vi "plugins_load.vi"(6 "Sub Panel":refnum<vi>, 7 "Plugin Chooser":refnum<vi>) -> (0 "error out":errorcluster, 1 "Plugins":T1(array[cluster]), 2 "Sub Panel Out":refnum<vi>, 3 "Plugin Chooser Out":refnum<vi>)   [LabVIEW 2015]
uses:
  red_tweezers_globals_INTERNAL_VOLATILE.vi
panel:
  out "file or folder exists?":bool
  out "Plugins Folder":path
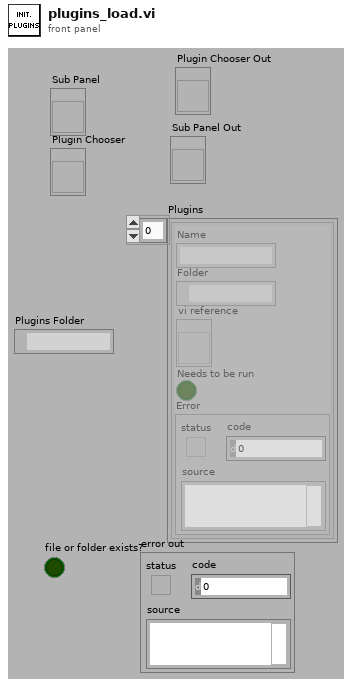
[diagram p1: front panel]
types:
  T1 = cluster{"Name":string, "Folder":path, "vi reference":refnum<vi>, "Needs to be run":bool, "Error":errorcluster}[]
  T2 = cluster{"Name":string, "Folder":path, "vi reference":refnum<vi>, "Needs to be run":bool, "Error":errorcluster}
  T3 = enum32{"Bad", "Idle", "Run top level", "Running"}
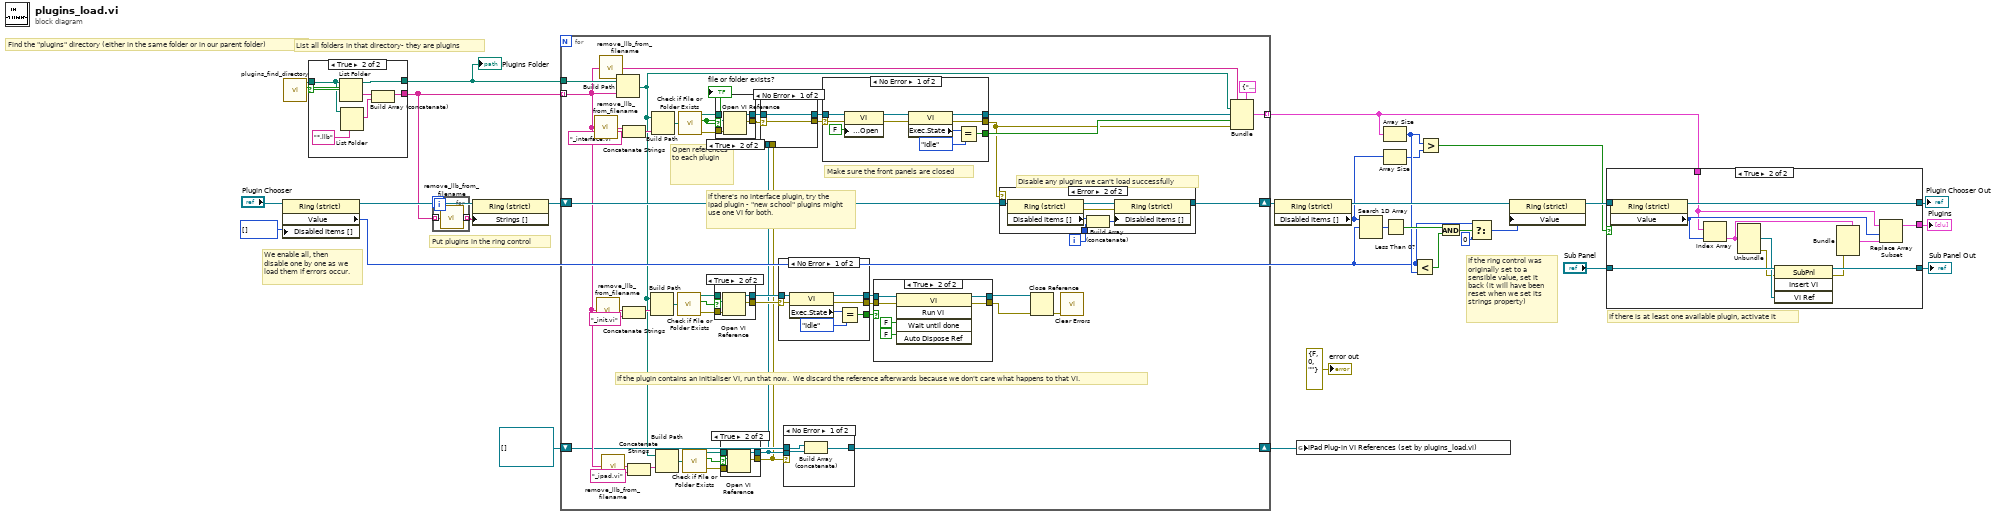
[diagram p0: block diagram]
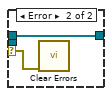
[diagram p4: hidden frame]
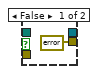
[diagram p5: hidden frame]
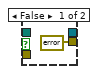
[diagram p7: hidden frame]
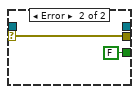
[diagram p8: hidden frame]
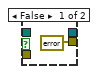
[diagram p10: hidden frame]
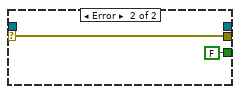
[diagram p11: hidden frame]
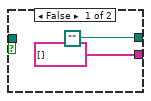
[diagram p12: hidden frame]
diagram:
  # "We enable all, then disable one by one as we load them if errors occur."
  # "If there is at least one available plugin, activate it"
  # "If the ring control was originally set to a sensible value, set it back (it will have been reset when we set its strings property)"
  # "Put plugins in the ring control"
  # "List all folders in that directory- they are plugins"
  # "Find the \"plugins\" directory (either in the same folder or in our parent folder)"
  n1 = property class="Ring (strict)"(reference="Plugin Chooser", "Disabled Items []"=i32[] []) -> (reference out=w25:refnum<vi>, "Value"=w4:u16)  [unwired: 1 in, 1 out]
  n2 = call "plugins_find_directory.vi"() -> ("file or folder exists?"=w30:bool, "dup path"=w31:path)  [unwired: 6 in]
  n3 = case shown="True" w30 {
    tunnel: w31 -> [_ w38]
    tunnel: [string[] [] ("folder names") w35] -> w9
    tunnel: [path "" w39] -> w29
    frame False {
    }
    frame True {
      n4 = List Folder(path=w38) -> (path out=w39:path, folder names=w36:string[])  [unwired: 3 in, 2 out]
      n5 = List Folder(path=w38, pattern="*.llb") -> (filenames=w34:string[])  [unwired: 2 in, 3 out]
      n6 = Build Array (concatenate)(w36, w34) -> (w35:string[])
    }
  }
  "Plugins Folder" <- w29
  n7 = for {
    tunnel: w9 -> [w41] mode=indexing
    tunnel: [w40] -> w8 mode=indexing
    n8 = call "remove_llb_from_filename.vi"("String"=w41) -> ("result string"=w40:string)
  }
  n9 = property class="Ring (strict)"(reference=w25, "Strings []"=w8) -> (reference out=w27:refnum<vi>)  [unwired: 1 in, 1 out]
  n10 = for {
    tunnel: w9 -> [w51] mode=indexing
    tunnel: w29 -> [w85]
    shift-right: [w80] -> w26
    shift-left: w27 -> [w81]
    tunnel: [w78] -> w19 mode=indexing
    shift-right: [w50] -> w2
    shift-left: refnum<vi>[] [] -> [w49]
    i -> [w82]
    # "if there's no interface plugin, try the ipad plugin - \"new school\" plugins might use one VI for both."
    # "If the plugin contains an initialiser VI, run that now.  We discard the reference afterwards because we don't care what happens to that VI."
    # "Open references to each plugin"
    # "Make sure the front panels are closed"
    # "Disable any plugins we can't load successfully"
    n11 = call "remove_llb_from_filename.vi"("String"=w51) -> ("result string"=w60:string)
    n12 = call "remove_llb_from_filename.vi"("String"=w51) -> ("result string"=w59:string)
    n13 = call "remove_llb_from_filename.vi"("String"=w51) -> ("result string"=w61:string)
    n14 = call "remove_llb_from_filename.vi"("String"=w51) -> ("result string"=w58:string)
    n15 = Build Path(base path=w85, name or relative path=w51) -> (appended path=w48:path)
    n16 = Concatenate Strings(w59, "_init.vi" ("string")) -> (w71:string)
    n17 = Concatenate Strings(w60, "_interface.vi" ("string")) -> (w90:string)
    n18 = Concatenate Strings(w58, "_ipad.vi" ("string")) -> (w54:string)
    n19 = Build Path(base path=w48, name or relative path=w71) -> (appended path=w63:path)
    n20 = Build Path(base path=w48, name or relative path=w90) -> (appended path=w88:path)
    n21 = Build Path(base path=w48, name or relative path=w54) -> (appended path=w57:path)
    n22 = call <vilib>:"Check if File or Folder Exists.vi"("path"=w63) -> ("error out"=w69:errorcluster, "file or folder exists?"=w75:bool, "dup path"=w72:path)  [unwired: 8 in]
    n23 = call <vilib>:"Check if File or Folder Exists.vi"("path"=w88) -> ("error out"=w83:errorcluster, "file or folder exists?"=w86:bool, "dup path"=w87:path)  [unwired: 8 in]
    "file or folder exists?" <- w86
    n24 = call <vilib>:"Check if File or Folder Exists.vi"("path"=w57) -> ("error out"=w56:errorcluster, "file or folder exists?"=w52:bool, "dup path"=w53:path)  [unwired: 8 in]
    n25 = case shown="True" w75 {
      tunnel: w72 -> [_ w117]
      tunnel: [_ w116] -> w73
      tunnel: [errorcluster {"status"=TRUE, "code"=0, "source"=""} ("error out") w115] -> w74
      tunnel: w69 -> [_ w114]
      frame False {
      }
      frame True {
        n26 = Open VI Reference(vi path=w117, error in (no error)=w114) -> (vi reference=w116:refnum<vi>, error out=w115:errorcluster)  [unwired: 4 in]
      }
    }
    n27 = case shown="True" w86 {
      tunnel: w87 -> [_ w139]
      tunnel: [_ w138] -> w46
      tunnel: [errorcluster {"status"=TRUE, "code"=0, "source"=""} ("error out") w137] -> w47
      tunnel: w83 -> [_ w136]
      frame False {
      }
      frame True {
        n28 = Open VI Reference(vi path=w139, error in (no error)=w136) -> (vi reference=w138:refnum<vi>, error out=w137:errorcluster)  [unwired: 4 in]
      }
    }
    n29 = case shown="True" w52 {
      tunnel: w53 -> [_ w104]
      tunnel: [_ w103] -> w44
      tunnel: [errorcluster {"status"=TRUE, "code"=0, "source"=""} ("error out") w102] -> w43
      tunnel: w56 -> [_ w101]
      frame False {
      }
      frame True {
        n30 = Open VI Reference(vi path=w104, error in (no error)=w101) -> (vi reference=w103:refnum<vi>, error out=w102:errorcluster)  [unwired: 4 in]
      }
    }
    n31 = case shown="No Error" w47 {
      selector: w47 -> [w91 _]
      tunnel: w46 -> [w92 _]
      tunnel: [w92 w94] -> w45
      tunnel: w44 -> [_ w94]
      tunnel: w43 -> [_ w93]
      tunnel: [w91 w93] -> w42
      frame No Error {
      }
      frame Error {
      }
    }
    n32 = case shown="No Error" w74 {
      selector: w74 -> [w119 w125]
      tunnel: w73 -> [w118 _]
      tunnel: [w124 _] -> w66
      tunnel: [w123 FALSE] -> w68
      tunnel: [w120 w125] -> w67
      frame No Error {
        n33 = property class="VI"(reference=w118, error in=w119) -> (reference out=w124:refnum<vi>, error out=w120:errorcluster, "Exec.State"=w122:T3)
        n34 = Equal?(x=w122, y=T3."Idle" ("Execution:State")) -> (x = y?=w123:bool)
      }
      frame Error {
      }
    }
    n35 = case shown="No Error" w43 {
      selector: w43 -> [_ w98]
      tunnel: w44 -> [w97 _]
      tunnel: [w96 w99] -> w50
      tunnel: w49 -> [w95 w99]
      frame No Error {
        n36 = Build Array (concatenate)(w95, w97) -> (w96:refnum<vi>[])
      }
      frame Error {
        n37 = call <vilib>:"Clear Errors.vi"("error in (no error)"=w98) -> ()  [unwired: 5 in, 2 out]
      }
    }
    n38 = case shown="No Error" w42 {
      selector: w42 -> [w144 w150]
      tunnel: w45 -> [w149 _]
      tunnel: [w146 _] -> w76
      tunnel: [w145 FALSE] -> w84
      tunnel: [w140 w150] -> w79
      frame No Error {
        n39 = property class="VI"(reference=w149, error in=w144, "Front Panel.Open"=FALSE ("Front Panel Window:Open")) -> (reference out=w147:refnum<vi>, error out=w143:errorcluster)
        n40 = property class="VI"(reference=w147, error in=w143) -> (reference out=w146:refnum<vi>, error out=w140:errorcluster, "Exec.State"=w142:T3)
        n41 = Equal?(x=w142, y=T3."Idle" ("Execution:State")) -> (x = y?=w145:bool)
      }
      frame Error {
      }
    }
    n42 = case shown="True" w68 {
      tunnel: w66 -> [w106 w112]
      tunnel: w67 -> [w105 w111]
      tunnel: [w106 w108] -> w65
      tunnel: [w105 w107] -> w64
      frame False {
      }
      frame True {
        n43 = invoke class="VI" method="Run VI"(reference=w112, error in=w111, "Wait until done"=FALSE ("Wait Until Done"), "Auto Dispose Ref"=FALSE ("Auto Dispose Reference")) -> (reference out=w108:refnum<vi>, error out=w107:errorcluster)  [unwired: 1 in, 3 out]
      }
    }
    n44 = case shown="Error" w79 {
      tunnel: w82 -> [_ w130]
      tunnel: w81 -> [w127 w129]
      tunnel: [w127 w128] -> w80
      frame No Error {
      }
      frame Error {
        n45 = property class="Ring (strict)"(reference=w129) -> (reference out=w134:refnum<vi>, error out=w133:errorcluster, "Disabled Items []"=w132:i32[])  [unwired: 1 in]
        n46 = Build Array (concatenate)(w132, w130) -> (w131:i32[])
        n47 = property class="Ring (strict)"(reference=w134, error in=w133, "Disabled Items []"=w131) -> (reference out=w128:refnum<vi>)  [unwired: 1 out]
      }
    }
    n48 = Close Reference(reference=w65, error in (no error)=w64) -> (error out=w62:errorcluster)
    n49 = call <vilib>:"Clear Errors.vi"("error in (no error)"=w62) -> ()  [unwired: 5 in, 2 out]
    n50 = Bundle(cluster=T2 {"Name"="", "Folder"=path "", "vi reference"=refnum, "Needs to be run"=FALSE, "Error"={"status"=FALSE, "code"=0, "source"=""}}, "Name"=w61, "Folder"=w48, "vi reference"=w76, "Needs to be run"=w84, "Error"=w79) -> (w78:T2)
  }
  n51 = property class="Ring (strict)"(reference=w26) -> (reference out=w24:refnum<vi>, "Disabled Items []"=w17:i32[])  [unwired: 1 in, 1 out]
  n52 = global write "red_tweezers_globals_INTERNAL_VOLATILE.vi" "iPad Plug-in VI References (set by plugins_load.vi)"(w2) -> ()
  n53 = Search 1D Array(1D array=w17, element=w4) -> (index of element=w23:i32)  [unwired: 1 in]
  n54 = Array Size(array=w17) -> (size(s)=w15:i32)
  n55 = Array Size(array=w19) -> (size(s)=w16:i32)
  n56 = Less Than 0?(x=w23) -> (x < 0?=w22:bool)
  n57 = Less?(x=w4, y=w16) -> (x < y?=w21:bool)
  n58 = Greater?(x=w16, y=w15) -> (0:w14:bool)
  n59 = And(x=w22, y=w21) -> (x .and. y?=w5:bool)
  n60 = Select(t=w4, s=w5, f=u16 0) -> (s? t:f=w6:u16)
  n61 = property class="Ring (strict)"(reference=w24, "Value"=w6) -> (reference out=w20:refnum<vi>)  [unwired: 1 in, 1 out]
  n62 = case shown="True" w14 {
    tunnel: w20 -> [w154 w166]
    tunnel: [w154 w165] -> w18
    tunnel: w19 -> [w153 w156]
    tunnel: "Sub Panel" -> [w152 w164]
    tunnel: [w152 w162] -> w11
    tunnel: [w153 w155] -> w12
    frame False {
    }
    frame True {
      n63 = property class="Ring (strict)"(reference=w166) -> (reference out=w165:refnum<vi>, "Value"=w158:u16)  [unwired: 1 in, 1 out]
      n64 = Index Array(array=w156, index=w158) -> (element=w160:T2)
      n65 = Unbundle(w160) -> ("vi reference"=w163:refnum<vi>, "Error"=w161:errorcluster)  [unwired: 3 out]
      n66 = invoke class="SubPnl" method="Insert VI"(reference=w164, error in=w161, "VI Ref"=w163) -> (reference out=w162:refnum<vi>, error out=w159:errorcluster)  [unwired: 1 in, 2 out]
      n67 = Bundle(cluster=w160, "Error"=w159) -> (w157:T2)  [unwired: 4 in]
      n68 = Replace Array Subset(array=w156, new element=w157, index=w158) -> (w155:T1)
    }
  }
  "Plugins" <- w12
  "Plugin Chooser Out" <- w18
  "Sub Panel Out" <- w11
  "error out" <- errorcluster {"status"=FALSE, "code"=0, "source"=""} ("error out")
